vi "to string.vi"(8 "error in":errorcluster, 11 "FPGA Module configuration in":refnum<class "FPGA Module configuration.lvclass">) -> (0 "error out":errorcluster, 1 "data":string, 2 "version":string, 3 "FPGA Module configuration out":refnum<class "FPGA Module configuration.lvclass">)   [LabVIEW 2017, in "FPGA Module configuration.lvclass"]
doc: "Provides an interface for saving a module configuration to a file or other serialized data source. It is recommended that all children of this class store data in two sets--data required for its own initialization, and any data required for parent initialization--and that each implementation uses the <b>Call Parent Method</b> primitive to serialize parent information."
uses:
  FPGA Module configuration.lvclass
  FPGA Module configuration.lvclass/FPGA Module configuration.ctl
  current version.vi
  <vilib>/NI/Tag Bus Module Framework/module configuration/TBM module configuration.lvclass
  fpga channel/FPGA Channel.lvclass
  <vilib>/NI/Configuration Framework/serializable configuration/NISE_CEF_serializable configuration.lvclass
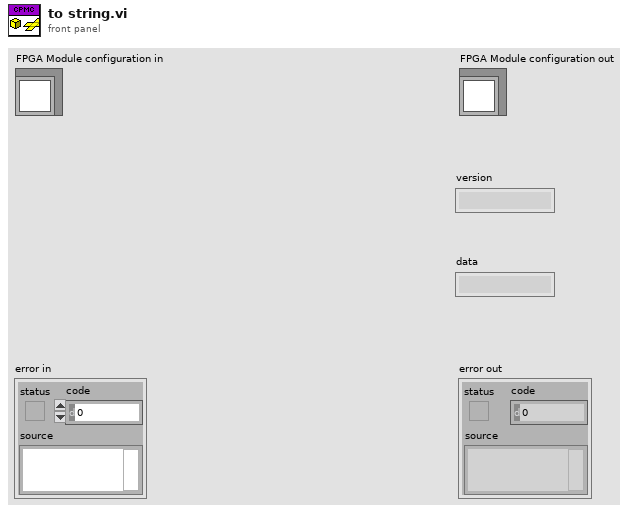
[diagram p1: front panel]
types:
  T1 = typedef "FPGA Module configuration.lvclass/Line.ctl" = cluster{"Channel":refnum<class "FPGA Channel.lvclass">}
  T2 = typedef "nirio_resource_hc.ctl" = tag
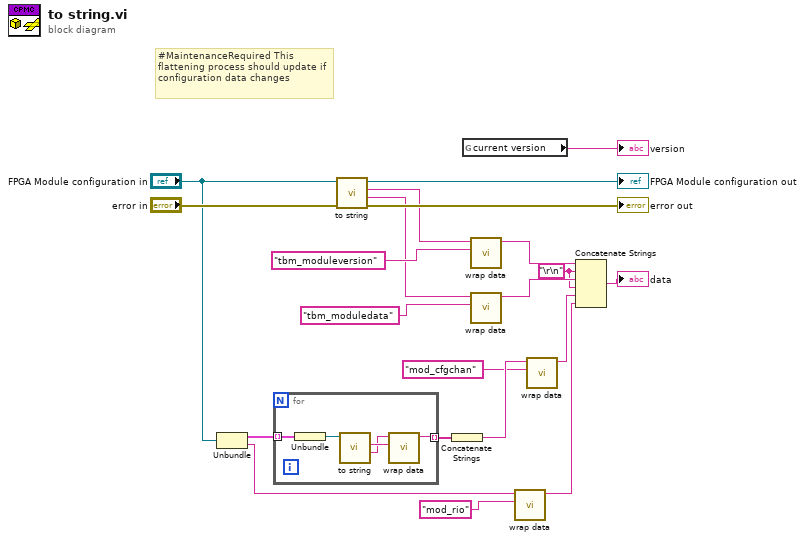
[diagram p0: block diagram]
diagram:
  w8 = "\r\n"
  # "#MaintenanceRequired This flattening process should update if configuration data changes"
  n1 = Unbundle("FPGA Module configuration in") -> (w7:T1[], w1:T2)
  n2 = for {
    tunnel: w7 -> [w26] mode=indexing
    tunnel: [w22] -> w6 mode=indexing
    n3 = Unbundle(w26) -> ("Channel"=w25:refnum<class "FPGA Channel.lvclass">)
    n4 = call-dynamic "to string.vi"("channel in"=w25) -> ("channel data"=w23:string, "identifier"=w24:string)  [unwired: 7 in, 2 out]
    n5 = call <vilib>:"wrap data.vi"("identifier"=w24, "data to wrap"=w23) -> ("wrapped data"=w22:string)  [unwired: 9 in]
  }
  n6 = call-parent "to string.vi"("error in"="error in", "module configuration in"="FPGA Module configuration in") -> ("error out"=→"error out":errorcluster, "data"=w12:string, "version"=w13:string, "module configuration out"=→"FPGA Module configuration out":refnum<class "FPGA Module configuration.lvclass">)  [unwired: 6 in]
  n7 = Concatenate Strings(w6) -> (w5:string)
  n8 = global read "current version.vi" "current version"() -> (→"version":string)
  n9 = call <vilib>:"wrap data.vi"("identifier"="tbm_moduleversion" ("additional identifier"), "data to wrap"=w13) -> ("wrapped data"=w15:string)  [unwired: 9 in]
  n10 = call <vilib>:"wrap data.vi"("identifier"="tbm_moduledata" ("additional identifier"), "data to wrap"=w12) -> ("wrapped data"=w14:string)  [unwired: 9 in]
  n11 = call <vilib>:"wrap data.vi"("identifier"="mod_rio", "data to wrap"=w1) -> ("wrapped data"=w3:string)  [unwired: 9 in]
  n12 = call <vilib>:"wrap data.vi"("identifier"="mod_cfgchan", "data to wrap"=w5) -> ("wrapped data"=w9:string)  [unwired: 9 in]
  n13 = Concatenate Strings(w15, w8, w14, w8, w9, w3) -> (→"data":string)
